vi "9.8.vi"() -> ()   [LabVIEW 2017]
uses:
  <vilib>/imath/engines/lvmath2/RunTimeEngine/Managers/WorkSpace/UID Generator.vi
  <vilib>/imath/engines/lvmath2/RunTimeEngine/ArithmeticOperatorToken/NIMS_ArithmeticOperator_power(S).vi
  <instcachedir>/0/NIMS_ArithmeticOperator_power(S)_86B1D76B77564424912EAFCCCC7488ED.lvgen/NIMS_ArithmeticOperator_power(S)_86B1D76B77564424912EAFCCCC7488ED_014.vi
  <vilib>/imathl/engines/lvmath/Functions/Error Handling/Create Error.vi
  <vilib>/imath/engines/lvmath2/RunTimeEngine/RunTimeType/NIMS_RunTimeType_From StrictType (excl LVString).vi
  <instcachedir>/0/NIMS_RunTimeType_From StrictType (excl LVString)_1019F277F0A747EDBCA0F6C52CA54500.lvgen/NIMS_RunTimeType_From StrictType (excl LVString)_1019F277F0A747EDBCA0F6C52CA54500_000.vi
  <vilib>/imath/engines/lvmath2/RunTimeEngine/LocalVariableDefStatement/MC_LocalVariableDefStatement_Display.vi
  <vilib>/imath/engines/lvmath2/RunTimeEngine/Managers/SymbolTable/Clear UID.vi
  <vilib>/imath/engines/lvmath2/RunTimeEngine/NodeEndStatement/NIMS_NodeEndStatement_Output.vi
  <instcachedir>/0/NIMS_NodeEndStatement_Output_53EC0D466D134D7ABD903AC30B43404B.lvgen/NIMS_NodeEndStatement_Output_53EC0D466D134D7ABD903AC30B43404B_001.vi
  <vilib>/imath/engines/lvmath2/RunTimeEngine/ErrorHandling/NIMS_Finalize Error.vi
  <vilib>/imath/engines/lvmath2/RunTimeEngine/Managers/SymbolTable/NIMS_WorkSpace.lvlib
panel:
  in  "bode":bool
  out "XY Graph":cluster{dbl[], dbl[]}(graph)
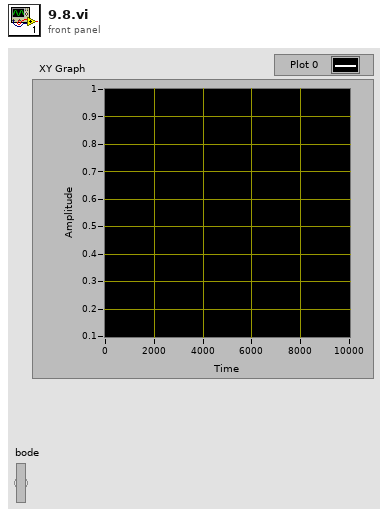
[diagram p1: front panel]
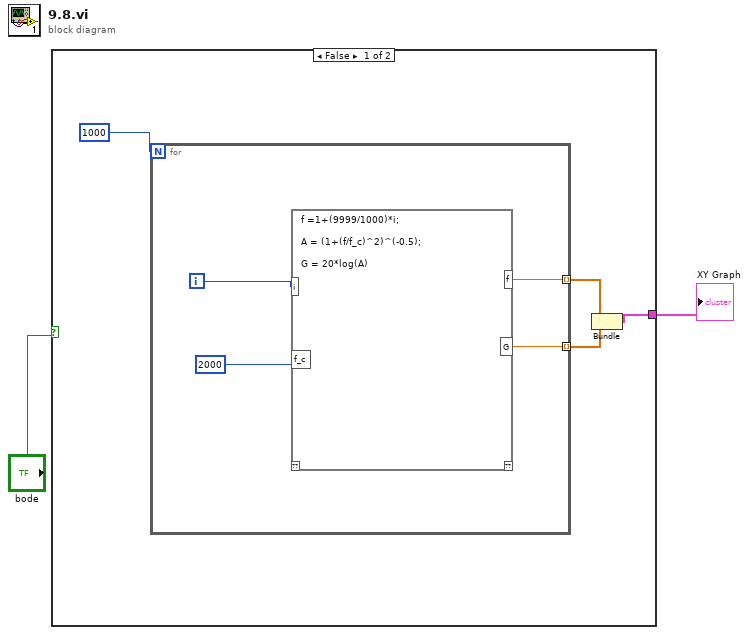
[diagram p0: block diagram]
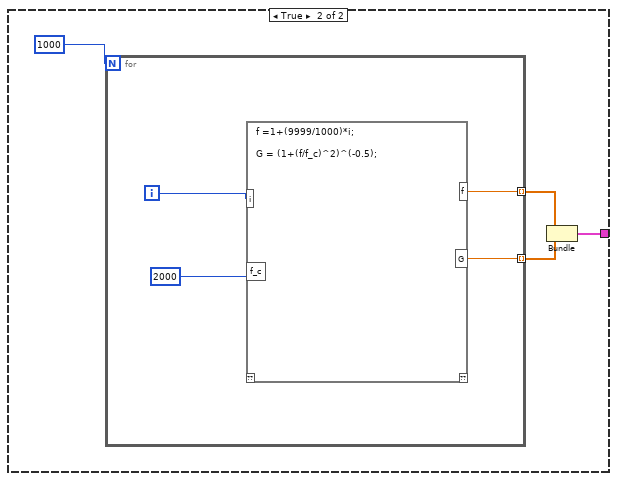
[diagram p2: hidden frame]
diagram:
  n1 = case shown="False" "bode" {
    tunnel: [w3 w87] -> w1
    frame False {
      n2 = for {
        N: 1000 -> [_]
        tunnel: [w8] -> w5 mode=indexing
        tunnel: [w7] -> w4 mode=indexing
        i -> [w10]
        n3 = mathscript code="f =1+(9999/1000)*i;\n\nA = (1+(f/f_c)^2)^(-0.5);\n\nG = 20*log(A)"("i"=w10, "f_c"=2000) -> ("f"=w8:dbl, "G"=w7:dbl)  [unwired: 1 in, 1 out]
      }
      n4 = Bundle(w5, w4) -> (w3:cluster{dbl[], dbl[]})  [unwired: 1 in]
    }
    frame True {
      n5 = for {
        N: 1000 -> [_]
        tunnel: [w92] -> w89 mode=indexing
        tunnel: [w91] -> w88 mode=indexing
        i -> [w94]
        n6 = mathscript code="f =1+(9999/1000)*i;\n\nG = (1+(f/f_c)^2)^(-0.5);"("i"=w94, "f_c"=2000) -> ("f"=w92:dbl, "G"=w91:dbl)  [unwired: 1 in, 1 out]
      }
      n7 = Bundle(w89, w88) -> (w87:cluster{dbl[], dbl[]})  [unwired: 1 in]
    }
  }
  "XY Graph" <- w1
